vi "Run Action_Do.vi"(8 "error in (no error)":errorcluster, 11 "Caraya Unit Test":refnum<class "Caraya Unit Test.lvclass">) -> (0 "error out":errorcluster, 1 "Success?":bool, 3 "Report Array":refnum<class "Report Data.lvclass">[](array[class]))   [LabVIEW 2020, in "ProjectBuilder.lvlib" / "Caraya Unit Test.lvclass"]
uses:
  Caraya Unit Test.lvclass
  C:/Current projects/WS/LV32.2020..ProjectBuilder/Class/Action/Project Action/Project Action.lvclass
  Data/Report Data/Report Data.lvclass
  Action/Project Action/Project Action.lvclass/Project Action.ctl
  Caraya Unit Test.lvclass/Caraya Unit Test.ctl
  Caraya Status Data/Caraya Status Data.lvclass/Caraya Status Data.ctl
  Caraya Status Data/Caraya Status Data.lvclass
  C:/Current projects/WS/LV32.2020..ProjectBuilder/Class/Data/Report Data/Report Data.lvclass
  PPL/Caraya.lvlibp/1abvi3w/vi.lib/addons/_JKI Toolkits/Caraya/run-tests/Run Test (ProjectRefnum).vi
  PPL/Caraya.lvlibp
  Action/Project Action/Project Action.lvclass
  ProjectBuilder.lvlib
  C:/Current projects/WS/LV32.2020..ProjectBuilder/Class/Caraya Unit Test/Caraya Status Data/Caraya Status Data.lvclass
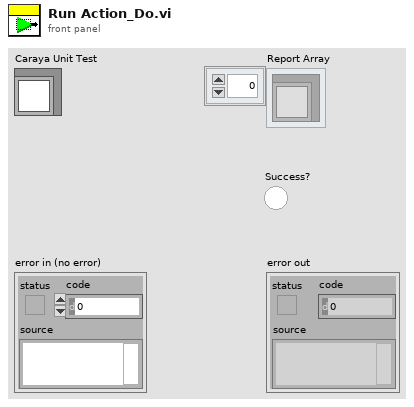
[diagram p1: front panel]
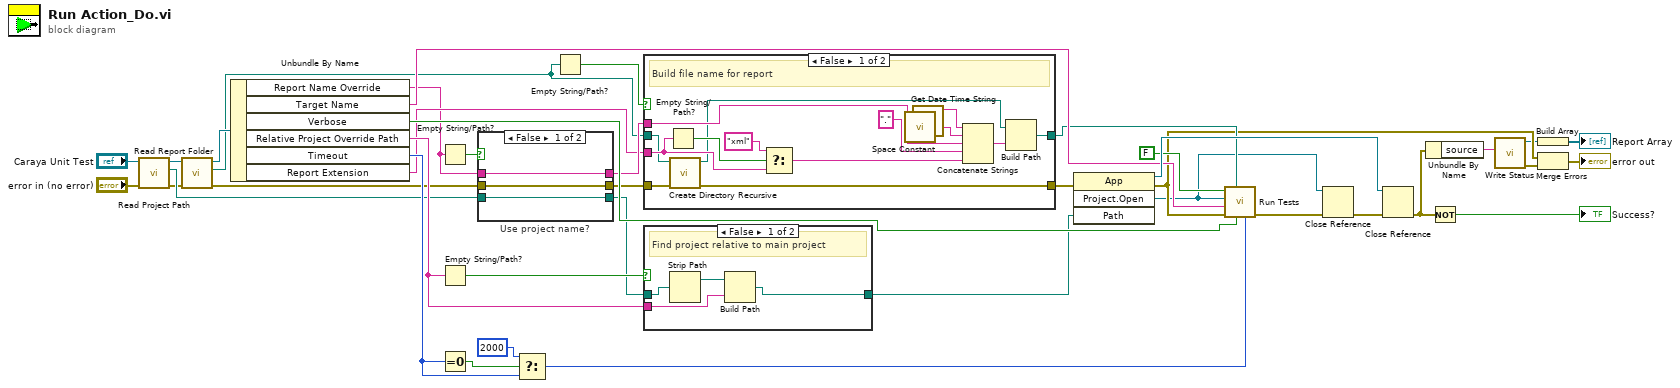
[diagram p0: block diagram]
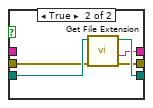
[diagram p2: hidden frame]
diagram:
  n1 = call "Read Project Path.vi"("error in (no error)"="error in (no error)", "Project Action in"="Caraya Unit Test") -> ("error out"=w18:errorcluster, "Project Path"=w24:path, "Project Action out"=w20:refnum<class "Caraya Unit Test.lvclass">)  [unwired: 7 in]
  n2 = call "Read Report Folder.vi"("error in (no error)"=w18, "Project Action in"=w20) -> ("error out"=w17:errorcluster, "Report Folder"=w14:path, "Project Action out"=w19:refnum<class "Caraya Unit Test.lvclass">)  [unwired: 7 in]
  n3 = Unbundle By Name(w19) -> ("Report Name Override"=w9:string, "Target Name"=w34:string, "Verbose"=w33:bool, "Relative Project Override Path"=w30:string, "Timeout"=w27:i32, "Report Extension"=w21:string)
  n4 = Empty String/Path?(string/path=w9) -> (empty?=w10:bool)
  n5 = Empty String/Path?(string/path=w30) -> (empty?=w32:bool)
  n6 = Equal To 0?(x=w27) -> (x = 0?=w28:bool)
  n7 = case "Use project name?" shown="False" w10 {
    tunnel: w24 -> [w42 w47]
    tunnel: [w42 w46] -> w23
    tunnel: [w41 w45] -> w22
    tunnel: w17 -> [w40 w44]
    tunnel: [w40 w43] -> w13
    tunnel: w9 -> [w41 _]
    frame False {
    }
    frame True {
      n8 = call <vilib>:"Get File Extension.vi"("error in (no error)"=w44, "file"=w47) -> ("error out"=w43:errorcluster, "filename without extension"=w45:string, "dup file"=w46:path)  [unwired: 5 in, 2 out]
    }
  }
  n9 = Select(t=2000, s=w28, f=w27) -> (s? t:f=w25:i32)
  n10 = Empty String/Path?(string/path=w14) -> (empty?=w16:bool)
  n11 = case shown="False" w16 {
    tunnel: w22 -> [w59 _]
    tunnel: w21 -> [w56 _]
    tunnel: [w48 w63] -> w15
    tunnel: w14 -> [w53 w63]
    tunnel: w13 -> [w52 w62]
    tunnel: [w51 w62] -> w12
    frame False {
      # "Build file name for report"
      n12 = Empty String/Path?(string/path=w56) -> (empty?=w57:bool)
      n13 = call <vilib>:"Create Directory Recursive.vi"("error in (no error)"=w52, "directory"=w53) -> ("error out"=w51:errorcluster, "directory copy"=w50:path)  [unwired: 3 in, 1 out]
      n14 = Select(t="xml", s=w57, f=w56) -> (s? t:f=w54:string)
      n15 = call <vilib>:"Space Constant.vi"() -> ("String"=w60:string)
      n16 = call "Get Date Time String.vi"() -> ("Time String"=w61:string)  [unwired: 11 in]
      n17 = Concatenate Strings(w61, w60, w59, "." ("string"), w54) -> (w49:string)
      n18 = Build Path(base path=w50, name or relative path=w49) -> (appended path=w48:path)
    }
    frame True {
      # "No report"
    }
  }
  n19 = case shown="False" w32 {
    tunnel: [w64 w68] -> w31
    tunnel: w23 -> [w67 w68]
    tunnel: w30 -> [w65 _]
    frame False {
      # "Find project relative to main project"
      n20 = Strip Path(path=w67) -> (stripped path=w66:path)  [unwired: 1 out]
      n21 = Build Path(base path=w66, name or relative path=w65) -> (appended path=w64:path)
    }
    frame True {
      # "No override"
    }
  }
  n22 = invoke class="App" method="Project.Open"(error in=w12, "Path"=w31) -> (reference out=w39:refnum<vi>, error out=w6:errorcluster, "Project:Open"=w1:refnum<vi>)  [unwired: 2 in, 1 out]
  n23 = call-poly "Run Tests.vi"("timeout (2000 ms)"=w25, "Verbose"=w33, "Report Path"=w15, "error in"=w6, "Virtual Folder (My Computer)"=w34, "Project Refnum"=w1, "Interactive (T)"=FALSE) -> ("error out"=w3:errorcluster)  [unwired: 4 in]
  n24 = Close Reference(reference=w1, error in (no error)=w3) -> (error out=w2:errorcluster)
  n25 = Close Reference(reference=w39, error in (no error)=w2) -> (error out=w29:errorcluster)
  n26 = Unbundle By Name(w29) -> ("source"=w8:string)
  n27 = Not(x=w29) -> (.not. x?=→"Success?":bool)
  n28 = call "Write Status.vi"("Status"=w8) -> ("error out"=w7:errorcluster, "Caraya Status Data out"=w4:refnum<class "Caraya Status Data.lvclass">)  [unwired: 9 in]
  n29 = Build Array(w4) -> (→"Report Array":refnum<class "Caraya Status Data.lvclass">[])
  n30 = Merge Errors(w6, w7) -> (→"error out":errorcluster)
